vi "SLL DE DI LV2 Global.vi"(6 "DI State Array":bool[](array[boolean]), 7 "Option":T2, 8 "error in (no error)":errorcluster, 9 "DI State":bool, 10 "DI Channel Name Array":T1[](array[typedef]), 11 "DI Channel Name":T1) -> (0 "error out":errorcluster, 1 "Array of all DIs":T1[](array[typedef]), 2 "Digital Array Status":bool[](array[boolean]), 3 "Digital Line Status":bool)   [LabVIEW 2013]
uses:
  Controls/SLL DE DI Global Options.ctl
  Controls/SLL DE List of Digital Inputs.ctl
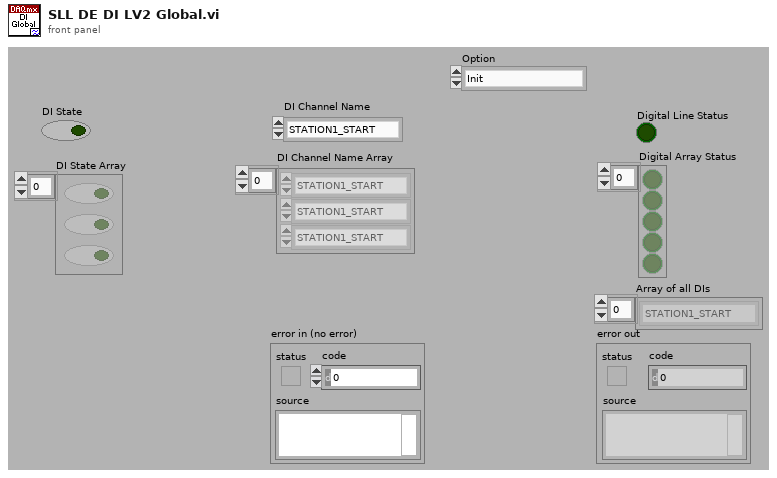
[diagram p1: front panel]
types:
  T1 = typedef "SLL DE List of Digital Inputs.ctl" = enum16{"STATION1_START", "STATION1_STOP", "STATION1_CLAMPED", "STATION1_TC_PASS", "STATION1_TC_FAIL", "STATION2_START", "STATION2_STOP", "STATION2_CLAMPED", "STATION2_TC_PASS", "STATION2_TC_FAIL", "STATION3_START", "STATION3_STOP", "STATION3_CLAMPED", "STATION3_TC_PASS", "STATION3_TC_FAIL", "STATION4_START", "STATION4_STOP", "STATION4_CLAMPED", "STATION4_TC_PASS", "STATION4_TC_FAIL"}
  T2 = typedef "SLL DE DI Global Options.ctl" = enum16{"Init", "Write Line", "Write Array", "Read Line", "Read Array", "Read Full Status", "Write Full Status"}
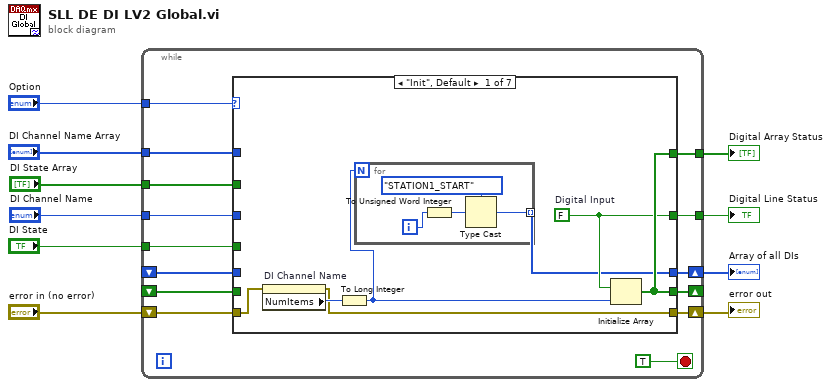
[diagram p0: block diagram]
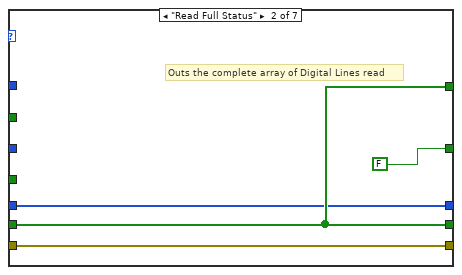
[diagram p2: hidden frame]
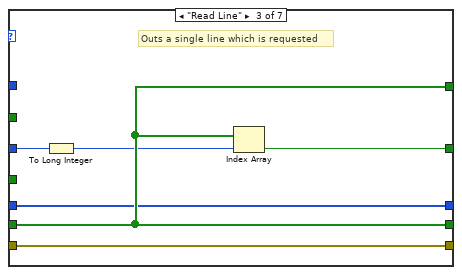
[diagram p3: hidden frame]
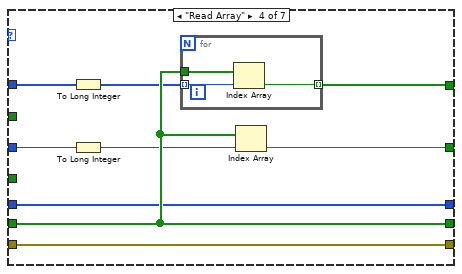
[diagram p4: hidden frame]
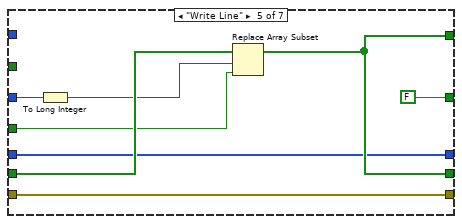
[diagram p5: hidden frame]
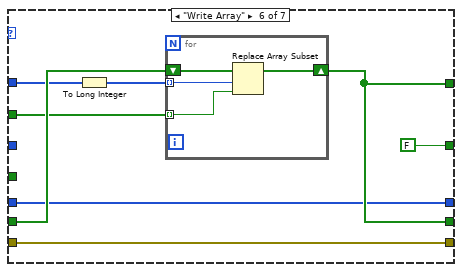
[diagram p6: hidden frame]
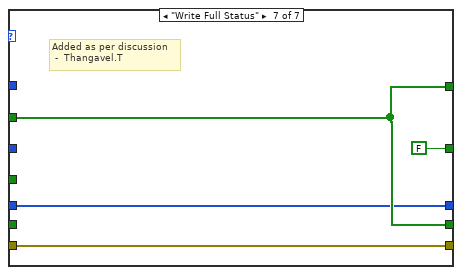
[diagram p7: hidden frame]
diagram:
  n1 = while {
    shift-right: [w23] -> _
    shift-left: _ -> [w22]
    tunnel: "DI Channel Name Array" -> [w21]
    tunnel: "DI Channel Name" -> [w20]
    tunnel: [w19] -> w8
    tunnel: [w18] -> w7
    shift-right: [w16] -> w5
    shift-left: "error in (no error)" -> [w17]
    tunnel: "DI State Array" -> [w15]
    tunnel: "DI State" -> [w14]
    tunnel: "Option" -> [w13]
    shift-right: [w12] -> w1
    shift-left: _ -> [w11]
    stop <- TRUE stop-if-true
    n2 = case shown="\"Init\", Default" w13 {
      tunnel: [w31 w39 w43 w51 w65 w73 w81] -> w23
      tunnel: w22 -> [_ w39 w43 w51 w62 w70 _]
      tunnel: w21 -> [_ _ _ w54 _ w68 _]
      tunnel: w20 -> [_ _ w45 w50 w60 _ _]
      tunnel: [w30 FALSE ("Digital Input") w44 w49 FALSE ("Digital Input") FALSE ("Digital Input") FALSE ("Digital Input")] -> w19
      tunnel: [w31 w39 w43 w53 w65 w73 w81] -> w18
      tunnel: w17 -> [w28 w37 w42 w52 w63 w71 w79]
      tunnel: [w27 w37 w42 w52 w63 w71 w79] -> w16
      tunnel: w15 -> [_ _ _ _ _ w69 w81]
      tunnel: w14 -> [_ _ _ _ w61 _ _]
      tunnel: [w25 w36 w40 w46 w58 w66 w80] -> w12
      tunnel: w11 -> [_ w36 w40 w46 w58 w66 w80]
      frame "Init", Default {
        w30 = FALSE  # Digital Input
        n3 = property on="DI Channel Name" class="Enum (strict)"(error in=w28) -> (error out=w27:errorcluster, "NumItems"=w29:u32)  [unwired: 1 in, 1 out]
        n4 = To Long Integer(number=w29) -> (32bit integer=w26:i32)
        n5 = for {
          N: w26 -> [_]
          tunnel: [w34] -> w25 mode=indexing
          i -> [w33]
          n6 = To Unsigned Word Integer(number=w33) -> (unsigned 16bit integer=w35:u16)
          n7 = Type Cast(type=SLL_DE_List_of_Digital_Inputs."STATION1_START" ("DI Channel Name"), x=w35) -> (*(type *) &x=w34:T1)
        }
        n8 = Initialize Array(w30, w26) -> (w31:bool[])
      }
      frame "Read Full Status" {
        # "Outs the complete array of Digital Lines read"
      }
      frame "Read Line" {
        # "Outs a single line which is requested"
        n9 = To Long Integer(number=w45) -> (32bit integer=w41:i32)
        n10 = Index Array(array=w43, index=w41) -> (element=w44:bool)
      }
      frame "Read Array" {
        n11 = To Long Integer(number=w54) -> (32bit integer=w47:i32[])
        n12 = To Long Integer(number=w50) -> (32bit integer=w48:i32)
        n13 = for {
          tunnel: w51 -> [w57]
          tunnel: w47 -> [w56] mode=indexing
          tunnel: [w55] -> w53 mode=indexing
          n14 = Index Array(array=w57, index=w56) -> (element=w55:bool)
        }
        n15 = Index Array(array=w51, index=w48) -> (element=w49:bool)
      }
      frame "Write Line" {
        n16 = To Long Integer(number=w60) -> (32bit integer=w59:i32)
        n17 = Replace Array Subset(array=w62, new element=w61, index=w59) -> (w65:bool[])
      }
      frame "Write Array" {
        n18 = To Long Integer(number=w68) -> (32bit integer=w67:i32[])
        n19 = for {
          tunnel: w69 -> [w75] mode=indexing
          shift-right: [w76] -> w73
          shift-left: w70 -> [w77]
          tunnel: w67 -> [w74] mode=indexing
          n20 = Replace Array Subset(array=w77, new element=w75, index=w74) -> (w76:bool[])
        }
      }
      frame "Write Full Status" {
        # "Added as per discussion\n -  Thangavel.T"
      }
    }
  }
  "error out" <- w5
  "Digital Line Status" <- w8
  "Digital Array Status" <- w7
  "Array of all DIs" <- w1
